vi "Climb_Teleop.vi"(11 "Joystick_In":T1) -> ()   [LabVIEW 2019]
uses:
  Globals/Climb_Globals.vi
  Subsystems/Climb/Climb_Cluster.ctl
  Utility_VIs/Joystick_Controls.ctl
panel:
  in  "fully_clamped(MAKE GLOBAL)":bool
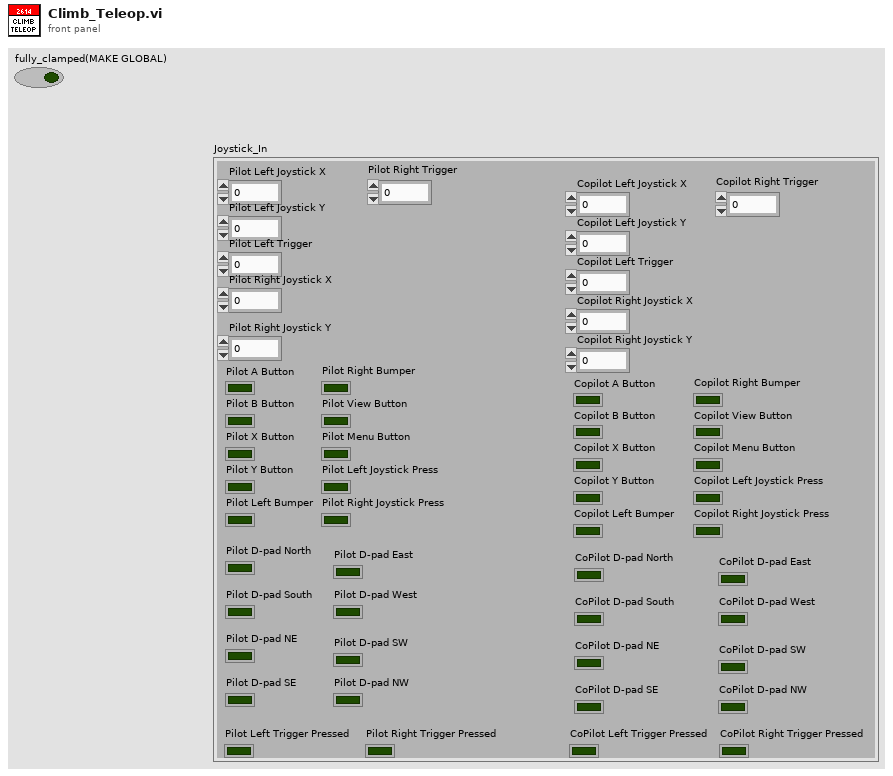
[diagram p1: front panel]
types:
  T1 = typedef "Joystick_Controls.ctl" = cluster{"Pilot Left Joystick X":dbl, "Pilot Left Joystick Y":dbl, "Pilot A Button":bool, "Pilot B Button":bool, "Pilot X Button":bool, "Pilot Y Button":bool, "Pilot Left Bumper":bool, "Pilot Right Bumper":bool, "Pilot View Button":bool, "Pilot Menu Button":bool, "Pilot Left Joystick Press":bool, "Pilot Right Joystick Press":bool, "Pilot Left Trigger":dbl, "Pilot Right Joystick X":dbl, "Pilot Right Joystick Y":dbl, "Pilot Right Trigger":dbl, "Copilot Left Joystick X":dbl, "Copilot Left Joystick Y":dbl, "Copilot A Button":bool, "Copilot B Button":bool, "Copilot X Button":bool, "Copilot Y Button":bool, "Copilot Left Bumper":bool, "Copilot Right Bumper":bool, "Copilot View Button":bool, "Copilot Menu Button":bool, "Copilot Left Joystick Press":bool, "Copilot Right Joystick Press":bool, "Copilot Left Trigger":dbl, "Copilot Right Joystick X":dbl, "Copilot Right Joystick Y":dbl, "Copilot Right Trigger":dbl, "Pilot D-pad North":bool, "Pilot D-pad South":bool, "Pilot D-pad East":bool, "Pilot D-pad West":bool, "Pilot D-pad NE ":bool, "Pilot D-pad SE":bool, "Pilot D-pad SW":bool, "Pilot D-pad NW":bool, "CoPilot D-pad North":bool, "CoPilot D-pad South":bool, "CoPilot D-pad East":bool, "CoPilot D-pad West":bool, "CoPilot D-pad NE":bool, "CoPilot D-pad SE":bool, "CoPilot D-pad SW":bool, "CoPilot D-pad NW":bool, "Pilot Left Trigger Pressed":bool, "Pilot Right Trigger Pressed":bool, "CoPilot Left Trigger Pressed":bool, "CoPilot Right Trigger Pressed":bool}
  T2 = typedef "Climb_Cluster.ctl" = cluster{"Control_State":enum16{"No-Op", "Extending", "Clamping", "Balancing", "Manual_Control"}, "Extend_Climber?":bool, "Clamp?":bool, "Balance?":bool, "Joint_Throttle":dbl, "LeadScrew_Throttle":dbl, "Control_Panel_Setpoint?":bool, "Auto-Balance":bool}
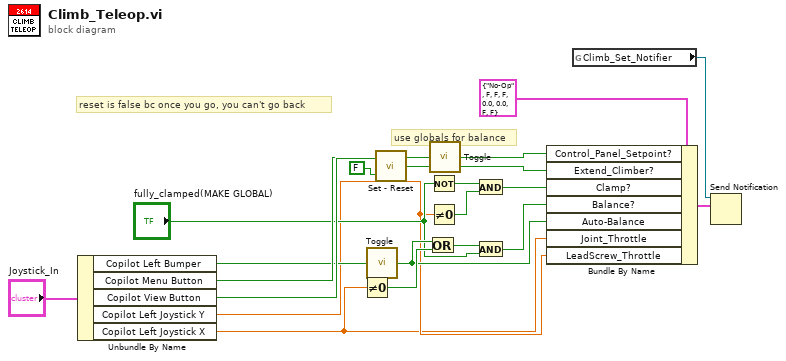
[diagram p0: block diagram]
diagram:
  # "use globals for balance"
  # "reset is false bc once you go, you can't go back"
  n1 = Unbundle By Name("Joystick_In") -> ("Copilot Left Bumper"=w11:bool, "Copilot Menu Button"=w12:bool, "Copilot View Button"=w15:bool, "Copilot Left Joystick Y"=w3:dbl, "Copilot Left Joystick X"=w1:dbl)
  n2 = Not Equal To 0?(x=w1) -> (x != 0?=w10:bool)
  n3 = call "Toggle.vi"("Boolean"=w11) -> ("Boolean Out"=w8:bool)
  n4 = call "Set - Reset.vi"("Reset"=FALSE, "Set"=w15) -> ("Output"=w14:bool)
  n5 = Or(x=w8, y=w10) -> (x .or. y?=w7:bool)
  n6 = Not(x="fully_clamped(MAKE GLOBAL)") -> (.not. x?=w5:bool)
  n7 = Not Equal To 0?(x=w3) -> (x != 0?=w4:bool)
  n8 = call "Toggle.vi"("Boolean"=w12) -> ("Boolean Out"=w13:bool)
  n9 = And(x=w5, y=w4) -> (x .and. y?=w2:bool)
  n10 = And(x=w7, y="fully_clamped(MAKE GLOBAL)") -> (x .and. y?=w9:bool)
  n11 = Bundle By Name(cluster=T2 {"Control_State"=enum."No-Op", "Extend_Climber?"=FALSE, "Clamp?"=FALSE, "Balance?"=FALSE, "Joint_Throttle"=0.0, "LeadScrew_Throttle"=0.0, "Control_Panel_Setpoint?"=FALSE, "Auto-Balance"=FALSE} ("notification"), "Control_Panel_Setpoint?"=w13, "Extend_Climber?"=w14, "Clamp?"=w2, "Balance?"=w9, "Auto-Balance"=w8, "Joint_Throttle"=w1, "LeadScrew_Throttle"=w3) -> (w17:T2)
  n12 = global read "Climb_Globals.vi" "Climb_Set_Notifier"() -> (w19:refnum<notifier>)
  n13 = Send Notification(notification=w17, notifier=w19) -> ()  [unwired: 1 in, 2 out]
